vi "Initialize MeasurementLink Session.vi"(7 "remote connection options":T2, 8 "error in":errorcluster, 9 "initialize and close session behavior":T1, 10 "session initialization parameters":T3, 11 "session factory in":refnum<class "ISession Factory.lvclass">) -> (0 "error out":errorcluster, 2 "session out":variant, 3 "session factory out":refnum<class "ISession Factory.lvclass">)   [LabVIEW 2021, in "NI Session Management Instrument.lvlib" / "ISession Factory.lvclass"]
doc: "Creates a new session using the provided <b>session initialization parameters</b>. If the session represents a remote session, <b>initialize and close session behavior</b> determines whether creating the local session creates a new session on the server or attaches to an existing session on the server."
uses:
  ISession Factory.lvclass
  Session Initialization Parameters.ctl
  Remote Connection Options.ctl
  Initialize and Close Session Behavior.ctl
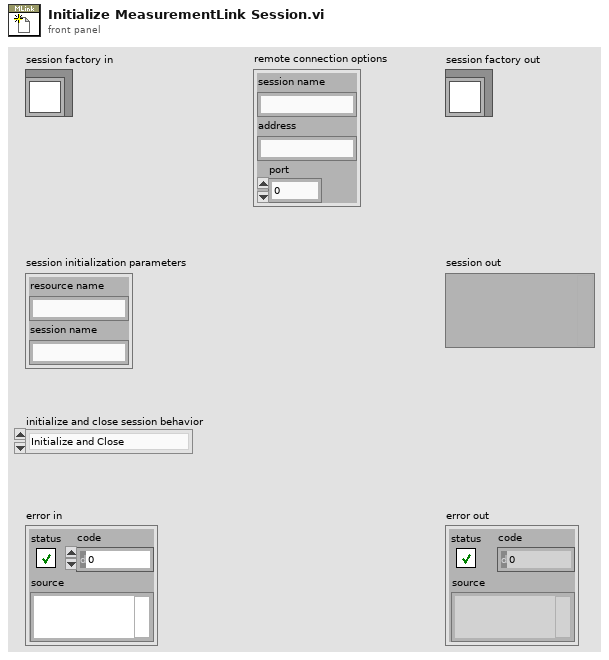
[diagram p1: front panel]
types:
  T1 = typedef "NI Session Management Instrument.lvlib/ISession Factory.lvclass/Initialize and Close Session Behavior.ctl" = enum16{"Initialize and Close", "Attach and Detach", "Initialize and Detach", "Attach and Close"}
  T2 = typedef "NI Session Management Instrument.lvlib/ISession Factory.lvclass/Remote Connection Options.ctl" = cluster{"session name":string, "address":string, "port":u32}
  T3 = typedef "NI Session Management Instrument.lvlib/ISession Factory.lvclass/Session Initialization Parameters.ctl" = cluster{"resource name":string, "session name":string}
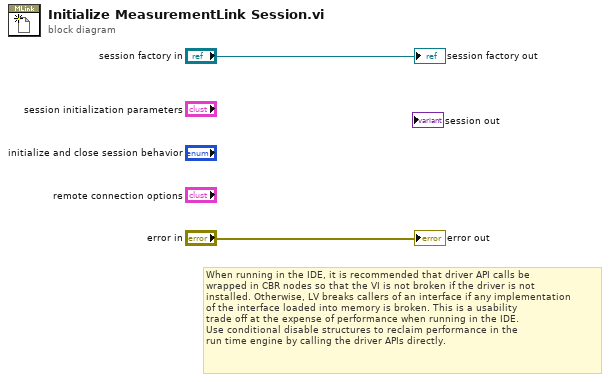
[diagram p0: block diagram]
diagram:
  # "When running in the IDE, it is recommended that driver API calls be \nwrapped in CBR nodes so that the VI is not broken if the driver is not \ninstalled. Otherwise, LV breaks callers of an interface if any implementation\nof the interface loaded into memory is broken. This is a usability\ntrade off at the expense of performance when running in the IDE.\nUse conditional disable structures to reclaim performance in the \nrun time engine by calling the driver APIs directly."
  "error out" <- "error in"
  "session factory out" <- "session factory in"
